vi "New.vi"(8 "error in (no error)":errorcluster, 10 "Listbox":refnum<vi>, 11 "String":refnum<vi>) -> (0 "error out":errorcluster, 3 "Handle out":refnum<class "Handle.lvclass">)   [LabVIEW 2021, in "Autocomplete Textbox.lvlib" / "Handle.lvclass"]
uses:
  Handle.lvclass
  ToMain UE.ctl
  ToMain UE action.ctl
  Handle.lvclass/Handle.ctl
  Autocomplete Textbox.lvlib
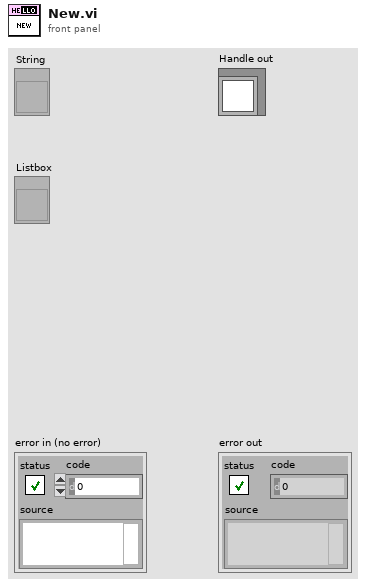
[diagram p1: front panel]
types:
  T1 = typedef "Autocomplete Textbox.lvlib/Handle.lvclass/ToMain UE.ctl" = cluster{"Type":T2, "data":variant}
  T2 = typedef "Autocomplete Textbox.lvlib/Handle.lvclass/ToMain UE action.ctl" = enum16{"New List", "Shutdown", "New Value", "Mouse Down (signal)"}
  T3 = enum32{"Invalid", "Standard", "Closed", "Hidden", "Minimized", "Maximized"}
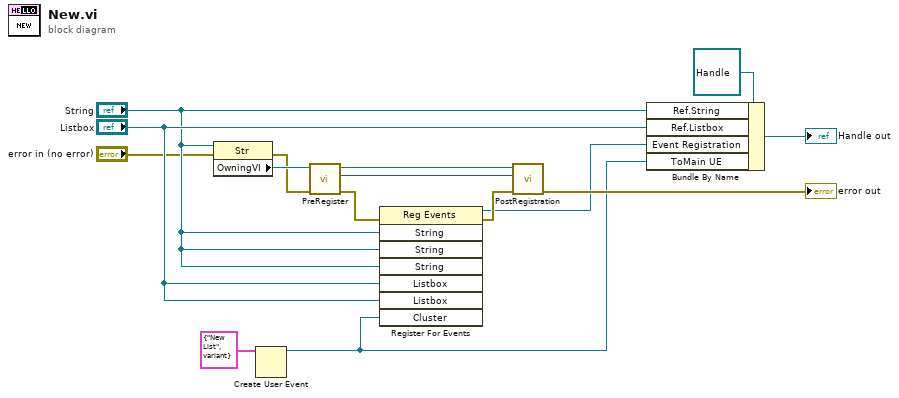
[diagram p0: block diagram]
diagram:
  n1 = property class="Str"(reference="String", error in="error in (no error)") -> (error out=w8:errorcluster, "OwningVI"=w9:refnum<vi>)  [unwired: 1 out]
  n2 = Create User Event(user event datatype=T1 {"Type"=enum."New List", "data"=variant} ("Cluster")) -> (user event=w2:refnum<user-event>)  [unwired: 1 in, 1 out]
  n3 = call "PreRegister.vi"("error in (no error)"=w8, "VI ref"=w9) -> ("error out"=w13:errorcluster, "state"=w4:T3, "VI ref"=w12:refnum<vi>)  [unwired: 7 in]
  n4 = register-events(error in=w13, "String", "String", "String", "Listbox", "Listbox", w2) -> (reference out=w1:refnum<event-registration>, error out=w11:errorcluster)  [unwired: 1 in]
  n5 = call "PostRegistration.vi"("error in (no error)"=w11, "state"=w4, "VI ref"=w12) -> ("error out"=→"error out":errorcluster)  [unwired: 7 in, 1 out]
  n6 = Bundle By Name(cluster=refnum<class "Handle.lvclass"> refnum ("Handle out"), "Ref.String"="String", "Ref.Listbox"="Listbox", "Event Registration"=w1, "ToMain UE"=w2) -> (→"Handle out":refnum<class "Handle.lvclass">)
